vi "GetstatusDEST.vi"(10 "error in (no error)":errorcluster, 11 "new reference":refnum<k24>) -> (0 "Dest":dbl[](array[numeric]), 2 "error out":errorcluster, 3 "reference out":refnum<k24>)   [LabVIEW 2017]
uses:
  C:/KMotion434/KMotion/Release/KMotion_dotNet.dll
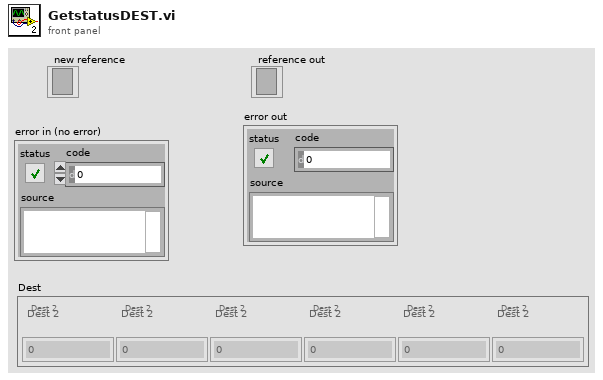
[diagram p1: front panel]
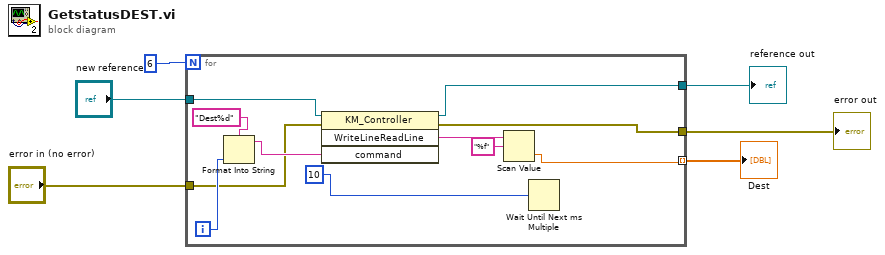
[diagram p0: block diagram]
diagram:
  n1 = for {
    N: 6 -> [_]
    tunnel: [w11] -> w5 mode=indexing
    tunnel: "new reference" -> [w10]
    tunnel: [w9] -> w3
    tunnel: "error in (no error)" -> [w8]
    tunnel: [w7] -> w1
    i -> [w12]
    n2 = Format Into String(format string="Dest%d" ("command"), w12) -> (resulting string=w13:string)  [unwired: 2 in, 1 out]
    n3 = invoke class="KM_Controller" method="WriteLineReadLine"(reference=w10, error in=w8, "command"=w13) -> (reference out=w9:refnum<k24>, error out=w7:errorcluster, "WriteLineReadLine"=w17:string)  [unwired: 1 in, 1 out]
    n4 = Scan Value(string=w17, format string="%f") -> (value=w11:dbl)  [unwired: 1 in, 1 out]
    n5 = Wait Until Next ms Multiple(millisecond multiple=u32 10) -> ()  [unwired: 1 out]
  }
  "Dest" <- w5
  "reference out" <- w3
  "error out" <- w1
